vi "Constant Elements Slices.vi"(4 "Array Stop (NaN: last)":dbl=nan, 6 "Array Start (NaN: first)":dbl=nan, 8 "Error In":errorcluster, 10 "# Elements":i32=1, 11 "Sorted Array in":dbl[](array[numeric])) -> (0 "Error Out":errorcluster, 1 "Valid Number?":bool, 2 "Bin Widths":dbl[](array[numeric]), 3 "Bin Bounds":dbl[](array[numeric]))   [LabVIEW 2021, in "Arrays.lvlib"]
doc: "Slices an array into parts containing a constant number of elements."
uses:
  967418b9-862b-45b2-a879-765d1ce128bf.vi
  c804f721-b7c3-42ba-912a-025f87f57916.vi
  967418b9-862b-45b2-a879-765d1ce128bf.vi/8a80743f-1319-44c8-96b0-3ef8fc688731.vi
  967418b9-862b-45b2-a879-765d1ce128bf.vi/931f4f8f-d8c6-4056-833f-5c8fe97b24b9.vi
  Arrays.lvlib
panel:
  # "see the AlliGator License on the block diagram (Ctrl+E or Window:Show Block Diagram)"
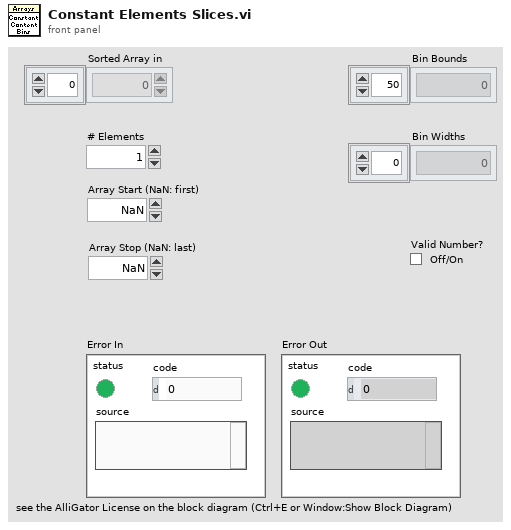
[diagram p1: front panel]
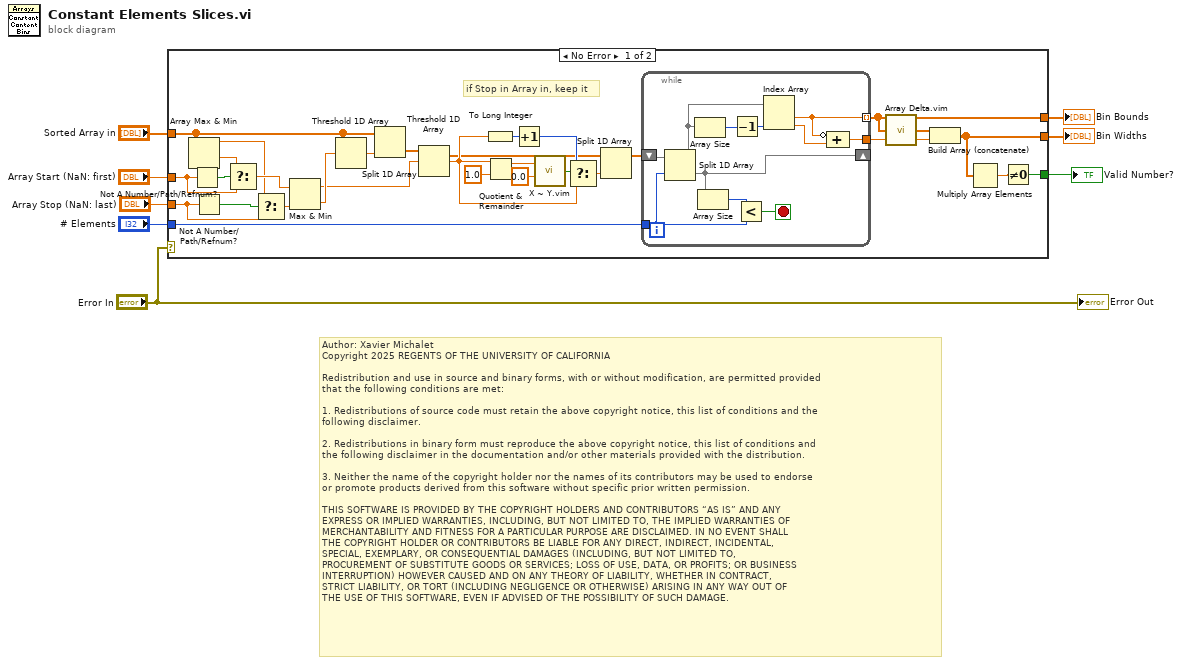
[diagram p0: block diagram]
diagram:
  # "Author: Xavier Michalet\nCopyright 2025 REGENTS OF THE UNIVERSITY OF CALIFORNIA\n\nRedistribution and use in source and binary forms, with or without modification, are permitted provided\nthat the following conditions are met:\n\n1. Redistributions of source code must retain the above copyright notice, this list of conditions and the\nfollowing disclaimer.\n\n2. Redistributions in binary form must reproduce the above copyright notice, this list of conditions and\nthe following disclaimer in the documentation and/or other materials provided with the distribution.\n\n3. Neither the name of the copyright holder nor the names of its contributors may be used to endorse \nor promote products derived from this software without specific prior written permission.\n\nTHIS SOFTWARE IS PROVIDED BY THE COPYRIGHT HOLDERS AND CONTRIBUTORS “AS IS” AND ANY \nEXPRESS OR IMPLIED WARRANTIES, INCLUDING, BUT NOT LIMITED TO, THE IMPLIED WARRANTIES OF\nMERCHANTABILITY AND FITNESS FOR A PARTICULAR PURPOSE ARE DISCLAIMED. IN NO EVENT SHALL\nTHE COPYRIGHT HOLDER OR CONTRIBUTORS BE LIABLE FOR ANY DIRECT, INDIRECT, INCIDENTAL, \nSPECIAL, EXEMPLARY, OR CONSEQUENTIAL DAMAGES (INCLUDING, BUT NOT LIMITED TO, \nPROCUREMENT OF SUBSTITUTE GOODS OR SERVICES; LOSS OF USE, DATA, OR PROFITS; OR BUSINESS\nINTERRUPTION) HOWEVER CAUSED AND ON ANY THEORY OF LIABILITY, WHETHER IN CONTRACT, \nSTRICT LIABILITY, OR TORT (INCLUDING NEGLIGENCE OR OTHERWISE) ARISING IN ANY WAY OUT OF\nTHE USE OF THIS SOFTWARE, EVEN IF ADVISED OF THE POSSIBILITY OF SUCH DAMAGE."
  n1 = case shown="No Error" "Error In" {
    tunnel: "# Elements" -> [w37 _]
    tunnel: "Sorted Array in" -> [w17 _]
    tunnel: "Array Start (NaN: first)" -> [w13 _]
    tunnel: "Array Stop (NaN: last)" -> [w9 _]
    tunnel: [w24 _] -> w4
    tunnel: [w21 _] -> w3
    tunnel: [w19 _] -> w2
    frame No Error {
      # "if Stop in Array in, keep it"
      n2 = Array Max & Min(array=w17) -> (max value=w11:dbl, min value=w15:dbl)  [unwired: 2 out]
      n3 = Not A Number/Path/Refnum?(number/path/refnum=w13) -> (NaN/Path/Refnum?=w16:bool)
      n4 = Not A Number/Path/Refnum?(number/path/refnum=w9) -> (NaN/Path/Refnum?=w12:bool)
      n5 = Select(t=w15, s=w16, f=w13) -> (s? t:f=w14:dbl)
      n6 = Select(t=w11, s=w12, f=w9) -> (s? t:f=w10:dbl)
      n7 = Max & Min(x=w14, y=w10) -> (max(x,y)=w35:dbl, min(x,y)=w36:dbl)
      n8 = Threshold 1D Array(2:w36, 3:w17) -> (0:w34:dbl)  [unwired: 1 in]
      n9 = Split 1D Array(array=w17, index=w34) -> (second subarray=w26:dbl[])  [unwired: 1 out]
      n10 = Threshold 1D Array(2:w35, 3:w26) -> (0:w28:dbl)  [unwired: 1 in]
      n11 = To Long Integer(number=w28) -> (32bit integer=w30:i32)
      n12 = Quotient & Remainder(x=w28, y=1.0) -> (x-y*floor(x/y)=w18:dbl)  [unwired: 1 out]
      n13 = Increment(x=w30) -> (x+1=w29:i32)
      n14 = call "X ~ Y.vim"("X"=w18, "Y"=0.0) -> ("X ~= Y?"=w31:bool)  [unwired: 13 in]
      n15 = Select(t=w29, s=w31, f=w28) -> (s? t:f=w27:dbl)
      n16 = Split 1D Array(array=w26, index=w27) -> (first subarray=w25:dbl[])  [unwired: 1 out]
      n17 = while {
        shift-right: [w47] -> _
        shift-left: w25 -> [w48]
        tunnel: w37 -> [w45]
        tunnel: [w40] -> w24 mode=indexing
        tunnel: [w38] -> w22
        stop <- w44 stop-if-true
        n18 = Split 1D Array(array=w48, index=w45) -> (first subarray=w43:dbl[], second subarray=w47:dbl[])
        n19 = Array Size(array=w43) -> (size(s)=w42:i32)
        n20 = Array Size(array=w47) -> (size(s)=w46:i32)
        n21 = Decrement(x=w42) -> (x-1=w41:i32)
        n22 = Less?(x=w46, y=w45) -> (x < y?=w44:bool)
        n23 = Index Array(array=w43, index #2=w41) -> (element #1=w40:dbl, element #2=w39:dbl)  [unwired: 1 in]
        n24 = Compound Arithmetic op=ADD(invert w40, w39) -> (w38:dbl)
      }
      n25 = call "Array Delta.vim"("A"=w24) -> ("A[i+1]-A[i]"=w23:dbl[])  [unwired: 8 in]
      n26 = Build Array (concatenate)(w23, w22) -> (w21:dbl[])
      n27 = Multiply Array Elements(1:w21) -> (0:w20:dbl)
      n28 = Not Equal To 0?(x=w20) -> (x != 0?=w19:bool)
    }
    frame Error {
    }
  }
  "Valid Number?" <- w2
  "Bin Widths" <- w3
  "Bin Bounds" <- w4
  "Error Out" <- "Error In"
